vi "WPI_DashboardLog NetworkTables.vi"(8 "Occasional DB Data":T1, 9 "Frequent DB Data":T2, 11 "NT Data Values":T7(array[cluster])) -> ()   [LabVIEW 2017]
uses:
  <vilib>/Rock Robotics/Network Tables/Protocol Operations.ctl
  <vilib>/Rock Robotics/Network Tables/Field Data.ctl
  <vilib>/Rock Robotics/Network Tables/Field Type.ctl
  <vilib>/Rock Robotics/Network Tables/Sequence.ctl
  <vilib>/Rock Robotics/Network Tables/Make Table Operation.ctl
  <vilib>/Rock Robotics/WPI/Dashboard/WPI_DashboardLogging Global.vi
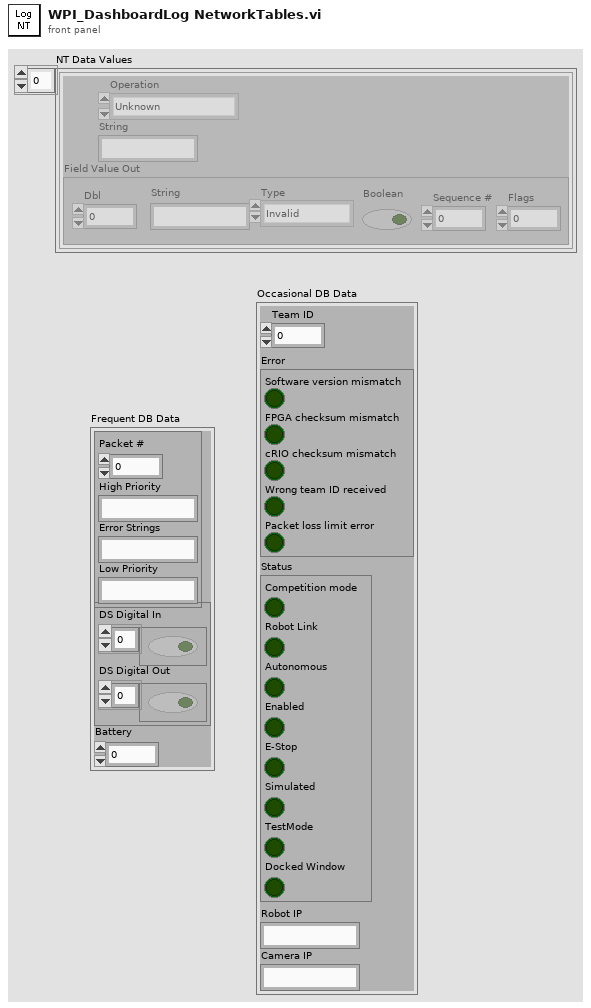
[diagram p1: front panel]
types:
  T1 = cluster{"Team ID":u16, "Error":cluster{"Software version mismatch":bool, "FPGA checksum mismatch":bool, "cRIO checksum mismatch":bool, "Wrong team ID received":bool, "Packet loss limit error":bool}, "Status":cluster{"Competition mode":bool, "Robot Link":bool, "Autonomous":bool, "Enabled":bool, "E-Stop":bool, "Simulated":bool, "TestMode":bool, "Docked Window":bool}, "Robot IP":string, "Camera IP":string}
  T2 = cluster{cluster{"Packet #":u8, "High Priority":string, "Error Strings":string, "Low Priority":string}, cluster{"DS Digital In":bool[], "DS Digital Out":bool[]}, "Battery":sgl}
  T3 = typedef "Protocol Operations.ctl" = enum16{"Unknown", "Keep Alive", "Client Hello", "Version not supported", "Server Hello Complete", "Assign", "Update", "No Op", "Server Hello", "Client Hello Complete", "Update Flags", "Delete Entry", "Delete All", "RPC Exec", "RPC Response"}
  T4 = typedef "Field Data.ctl" = cluster{"Dbl":dbl, "String":string, "Type":T5, "Boolean":bool, "Sequence #":T6, "Flags":u8}
  T5 = typedef "Field Type.ctl" = enum8{"Invalid", "Bool", "Numeric", "String", "Raw", "Boolean Array", "Numeric Array", "String Array", "RPC"}
  T6 = typedef "Sequence.ctl" = u16
  T7 = cluster{"Operation":T3, "String":string, "Field Value Out":T4}[]
  T8 = cluster{"size":u8, "tag":u8, "Version":cluster{"unsigned byte array[0]":u8, "unsigned byte array[1]":u8, "unsigned byte array[2]":u8, "unsigned byte array[3]":u8, "unsigned byte array[4]":u8, "unsigned byte array[5]":u8, "unsigned byte array[6]":u8, "unsigned byte array[7]":u8, "unsigned byte array[8]":u8, "unsigned byte array[9]":u8, "unsigned byte array[10]":u8}, "numPlayers":i8, "flags":u32, "floorClipPlane":cluster{"x":sgl, "y":sgl, "z":sgl, "w":sgl}, "Gravity Normal":cluster{"x":sgl, "y":sgl, "z":sgl}, "size":u8, "tag":u8, "Extra Data":cluster{"TrackingState":cluster{"TrackingState[0]":u8, "TrackingState[1]":u8, "TrackingState[2]":u8, "TrackingState[3]":u8, "TrackingState[4]":u8, "TrackingState[5]":u8, "TrackingState[6]":u8, "TrackingState[7]":u8, "TrackingState[8]":u8, "TrackingState[9]":u8, "TrackingState[10]":u8, "TrackingState[11]":u8, "TrackingState[12]":u8, "TrackingState[13]":u8, "TrackingState[14]":u8, "TrackingState[15]":u8, "TrackingState[16]":u8, "TrackingState[17]":u8, "TrackingState[18]":u8, "TrackingState[19]":u8}, "Position":cluster{"x":sgl, "y":sgl, "z":sgl}, "Quality":u32, "TrackState":enum32{"NotTracked", "PositionOnly", "Tracked"}}, "size":u8, "tag":u8, "Vertices":cluster{"Vertices[0]":cluster{"x":sgl, "y":sgl, "z":sgl}, "Vertices[1]":cluster{"x":sgl, "y":sgl, "z":sgl}, "Vertices[2]":cluster{"x":sgl, "y":sgl, "z":sgl}, "Vertices[3]":cluster{"x":sgl, "y":sgl, "z":sgl}, "Vertices[4]":cluster{"x":sgl, "y":sgl, "z":sgl}, "Vertices[5]":cluster{"x":sgl, "y":sgl, "z":sgl}, "Vertices[6]":cluster{"x":sgl, "y":sgl, "z":sgl}, "Vertices[7]":cluster{"x":sgl, "y":sgl, "z":sgl}, "Vertices[8]":cluster{"x":sgl, "y":sgl, "z":sgl}, "Vertices[9]":cluster{"x":sgl, "y":sgl, "z":sgl}, "Vertices[10]":cluster{"x":sgl, "y":sgl, "z":sgl}, "Vertices[11]":cluster{"x":sgl, "y":sgl, "z":sgl}, "Vertices[12]":cluster{"x":sgl, "y":sgl, "z":sgl}, "Vertices[13]":cluster{"x":sgl, "y":sgl, "z":sgl}, "Vertices[14]":cluster{"x":sgl, "y":sgl, "z":sgl}, "Vertices[15]":cluster{"x":sgl, "y":sgl, "z":sgl}, "Vertices[16]":cluster{"x":sgl, "y":sgl, "z":sgl}, "Vertices[17]":cluster{"x":sgl, "y":sgl, "z":sgl}, "Vertices[18]":cluster{"x":sgl, "y":sgl, "z":sgl}, "Vertices[19]":cluster{"x":sgl, "y":sgl, "z":sgl}}, "size":u8, "tag":u8, "Joystick":cluster{"axis 1":i8, "axis 2":i8, "axis 3":i8, "axis 4":i8, "axis 5":i8, "axis 6":i8, "Buttons":u16}, "Joystick 2":cluster{"axis 1":i8, "axis 2":i8, "axis 3":i8, "axis 4":i8, "axis 5":i8, "axis 6":i8, "Buttons":u16}, "size":u8, "tag":u8, "Custom Data":string}[]
  T9 = typedef "Make Table Operation.ctl" = enum16{"Get or Add Field", "Get Field or Add Temp", "Replace Temp ID", "Get Field ID - No Add", "Get Table Field IDs", "Get Field ID Info", "Move Field to Temp", "Validate", "Remove Field", "Remove All"}
  T10 = enum16{"open", "replace", "create", "open or create", "replace or create", "replace or create with confirmation"}
  T11 = cluster{"Operation":T3, "Name":string, "Field Value":T4}[]
  T12 = cluster{cluster{"High Priority":string, "Error Strings":string, "Low Priority":string}, cluster{u8, u8}, "Battery":sgl}
  T13 = cluster{"Team ID":u16, "Error":cluster{"Software version mismatch":bool, "FPGA checksum mismatch":bool, "cRIO checksum mismatch":bool, "Wrong team ID received":bool, "Packet loss limit error":bool}, "Status":cluster{"Competition mode":bool, "Robot Link":bool, "Autonomous":bool, "Enabled":bool, "E-Stop":bool, "Simulated":bool, "TestMode":bool, "Docked Window":bool}, "Robot IP":string, "Camera IP":string}[]
  T14 = cluster{"Video 1":i32, "Video 2":i32, "Video 3":i32, "Video 4":i32}
  T15 = cluster{i32, "Video Frame #":cluster{"Video 1":i32, "Video 2":i32, "Video 3":i32, "Video 4":i32}, "Logged Data":cluster{cluster{"High Priority":string, "Error Strings":string, "Low Priority":string}, cluster{u8, u8}, "Battery":sgl}, "Updates out":cluster{"Operation":T3, "Name":string, "Field Value":T4}[], cluster{"Team ID":u16, "Error":cluster{"Software version mismatch":bool, "FPGA checksum mismatch":bool, "cRIO checksum mismatch":bool, "Wrong team ID received":bool, "Packet loss limit error":bool}, "Status":cluster{"Competition mode":bool, "Robot Link":bool, "Autonomous":bool, "Enabled":bool, "E-Stop":bool, "Simulated":bool, "TestMode":bool, "Docked Window":bool}, "Robot IP":string, "Camera IP":string}[], "Kinect Data":cluster{"size":u8, "tag":u8, "Version":cluster{"unsigned byte array[0]":u8, "unsigned byte array[1]":u8, "unsigned byte array[2]":u8, "unsigned byte array[3]":u8, "unsigned byte array[4]":u8, "unsigned byte array[5]":u8, "unsigned byte array[6]":u8, "unsigned byte array[7]":u8, "unsigned byte array[8]":u8, "unsigned byte array[9]":u8, "unsigned byte array[10]":u8}, "numPlayers":i8, "flags":u32, "floorClipPlane":cluster{"x":sgl, "y":sgl, "z":sgl, "w":sgl}, "Gravity Normal":cluster{"x":sgl, "y":sgl, "z":sgl}, "size":u8, "tag":u8, "Extra Data":cluster{"TrackingState":cluster{"TrackingState[0]":u8, "TrackingState[1]":u8, "TrackingState[2]":u8, "TrackingState[3]":u8, "TrackingState[4]":u8, "TrackingState[5]":u8, "TrackingState[6]":u8, "TrackingState[7]":u8, "TrackingState[8]":u8, "TrackingState[9]":u8, "TrackingState[10]":u8, "TrackingState[11]":u8, "TrackingState[12]":u8, "TrackingState[13]":u8, "TrackingState[14]":u8, "TrackingState[15]":u8, "TrackingState[16]":u8, "TrackingState[17]":u8, "TrackingState[18]":u8, "TrackingState[19]":u8}, "Position":cluster{"x":sgl, "y":sgl, "z":sgl}, "Quality":u32, "TrackState":enum32{"NotTracked", "PositionOnly", "Tracked"}}, "size":u8, "tag":u8, "Vertices":cluster{"Vertices[0]":cluster{"x":sgl, "y":sgl, "z":sgl}, "Vertices[1]":cluster{"x":sgl, "y":sgl, "z":sgl}, "Vertices[2]":cluster{"x":sgl, "y":sgl, "z":sgl}, "Vertices[3]":cluster{"x":sgl, "y":sgl, "z":sgl}, "Vertices[4]":cluster{"x":sgl, "y":sgl, "z":sgl}, "Vertices[5]":cluster{"x":sgl, "y":sgl, "z":sgl}, "Vertices[6]":cluster{"x":sgl, "y":sgl, "z":sgl}, "Vertices[7]":cluster{"x":sgl, "y":sgl, "z":sgl}, "Vertices[8]":cluster{"x":sgl, "y":sgl, "z":sgl}, "Vertices[9]":cluster{"x":sgl, "y":sgl, "z":sgl}, "Vertices[10]":cluster{"x":sgl, "y":sgl, "z":sgl}, "Vertices[11]":cluster{"x":sgl, "y":sgl, "z":sgl}, "Vertices[12]":cluster{"x":sgl, "y":sgl, "z":sgl}, "Vertices[13]":cluster{"x":sgl, "y":sgl, "z":sgl}, "Vertices[14]":cluster{"x":sgl, "y":sgl, "z":sgl}, "Vertices[15]":cluster{"x":sgl, "y":sgl, "z":sgl}, "Vertices[16]":cluster{"x":sgl, "y":sgl, "z":sgl}, "Vertices[17]":cluster{"x":sgl, "y":sgl, "z":sgl}, "Vertices[18]":cluster{"x":sgl, "y":sgl, "z":sgl}, "Vertices[19]":cluster{"x":sgl, "y":sgl, "z":sgl}}, "size":u8, "tag":u8, "Joystick":cluster{"axis 1":i8, "axis 2":i8, "axis 3":i8, "axis 4":i8, "axis 5":i8, "axis 6":i8, "Buttons":u16}, "Joystick 2":cluster{"axis 1":i8, "axis 2":i8, "axis 3":i8, "axis 4":i8, "axis 5":i8, "axis 6":i8, "Buttons":u16}, "size":u8, "tag":u8, "Custom Data":string}[]}
  T16 = typedef "Field ID.ctl" = i32
  T17 = cluster{"Operation":T3, "String":string, "Field Value Out":T4}
  T18 = cluster{"Version":i32, "Duration":i32, "seconds since 1Jan1904":timestamp, "Robot IP":string}
  T19 = cluster{i32, i32, "Logged Data":cluster{cluster{"High Priority":string, "Error Strings":string, "Low Priority":string}, cluster{u8, u8}, "Battery":sgl}, "Updates out":cluster{"Operation":T3, "Name":string, "Field Value":T4}[], cluster{"Team ID":u16, "Error":cluster{"Software version mismatch":bool, "FPGA checksum mismatch":bool, "cRIO checksum mismatch":bool, "Wrong team ID received":bool, "Packet loss limit error":bool}, "Status":cluster{"Competition mode":bool, "Robot Link":bool, "Autonomous":bool, "Enabled":bool, "E-Stop":bool, "Simulated":bool, "TestMode":bool, "Docked Window":bool}, "Robot IP":string, "Camera IP":string}[], "Kinect Data":cluster{"size":u8, "tag":u8, "Version":cluster{"unsigned byte array[0]":u8, "unsigned byte array[1]":u8, "unsigned byte array[2]":u8, "unsigned byte array[3]":u8, "unsigned byte array[4]":u8, "unsigned byte array[5]":u8, "unsigned byte array[6]":u8, "unsigned byte array[7]":u8, "unsigned byte array[8]":u8, "unsigned byte array[9]":u8, "unsigned byte array[10]":u8}, "numPlayers":i8, "flags":u32, "floorClipPlane":cluster{"x":sgl, "y":sgl, "z":sgl, "w":sgl}, "Gravity Normal":cluster{"x":sgl, "y":sgl, "z":sgl}, "size":u8, "tag":u8, "Extra Data":cluster{"TrackingState":cluster{"TrackingState[0]":u8, "TrackingState[1]":u8, "TrackingState[2]":u8, "TrackingState[3]":u8, "TrackingState[4]":u8, "TrackingState[5]":u8, "TrackingState[6]":u8, "TrackingState[7]":u8, "TrackingState[8]":u8, "TrackingState[9]":u8, "TrackingState[10]":u8, "TrackingState[11]":u8, "TrackingState[12]":u8, "TrackingState[13]":u8, "TrackingState[14]":u8, "TrackingState[15]":u8, "TrackingState[16]":u8, "TrackingState[17]":u8, "TrackingState[18]":u8, "TrackingState[19]":u8}, "Position":cluster{"x":sgl, "y":sgl, "z":sgl}, "Quality":u32, "TrackState":enum32{"NotTracked", "PositionOnly", "Tracked"}}, "size":u8, "tag":u8, "Vertices":cluster{"Vertices[0]":cluster{"x":sgl, "y":sgl, "z":sgl}, "Vertices[1]":cluster{"x":sgl, "y":sgl, "z":sgl}, "Vertices[2]":cluster{"x":sgl, "y":sgl, "z":sgl}, "Vertices[3]":cluster{"x":sgl, "y":sgl, "z":sgl}, "Vertices[4]":cluster{"x":sgl, "y":sgl, "z":sgl}, "Vertices[5]":cluster{"x":sgl, "y":sgl, "z":sgl}, "Vertices[6]":cluster{"x":sgl, "y":sgl, "z":sgl}, "Vertices[7]":cluster{"x":sgl, "y":sgl, "z":sgl}, "Vertices[8]":cluster{"x":sgl, "y":sgl, "z":sgl}, "Vertices[9]":cluster{"x":sgl, "y":sgl, "z":sgl}, "Vertices[10]":cluster{"x":sgl, "y":sgl, "z":sgl}, "Vertices[11]":cluster{"x":sgl, "y":sgl, "z":sgl}, "Vertices[12]":cluster{"x":sgl, "y":sgl, "z":sgl}, "Vertices[13]":cluster{"x":sgl, "y":sgl, "z":sgl}, "Vertices[14]":cluster{"x":sgl, "y":sgl, "z":sgl}, "Vertices[15]":cluster{"x":sgl, "y":sgl, "z":sgl}, "Vertices[16]":cluster{"x":sgl, "y":sgl, "z":sgl}, "Vertices[17]":cluster{"x":sgl, "y":sgl, "z":sgl}, "Vertices[18]":cluster{"x":sgl, "y":sgl, "z":sgl}, "Vertices[19]":cluster{"x":sgl, "y":sgl, "z":sgl}}, "size":u8, "tag":u8, "Joystick":cluster{"axis 1":i8, "axis 2":i8, "axis 3":i8, "axis 4":i8, "axis 5":i8, "axis 6":i8, "Buttons":u16}, "Joystick 2":cluster{"axis 1":i8, "axis 2":i8, "axis 3":i8, "axis 4":i8, "axis 5":i8, "axis 6":i8, "Buttons":u16}, "size":u8, "tag":u8, "Custom Data":string}[]}
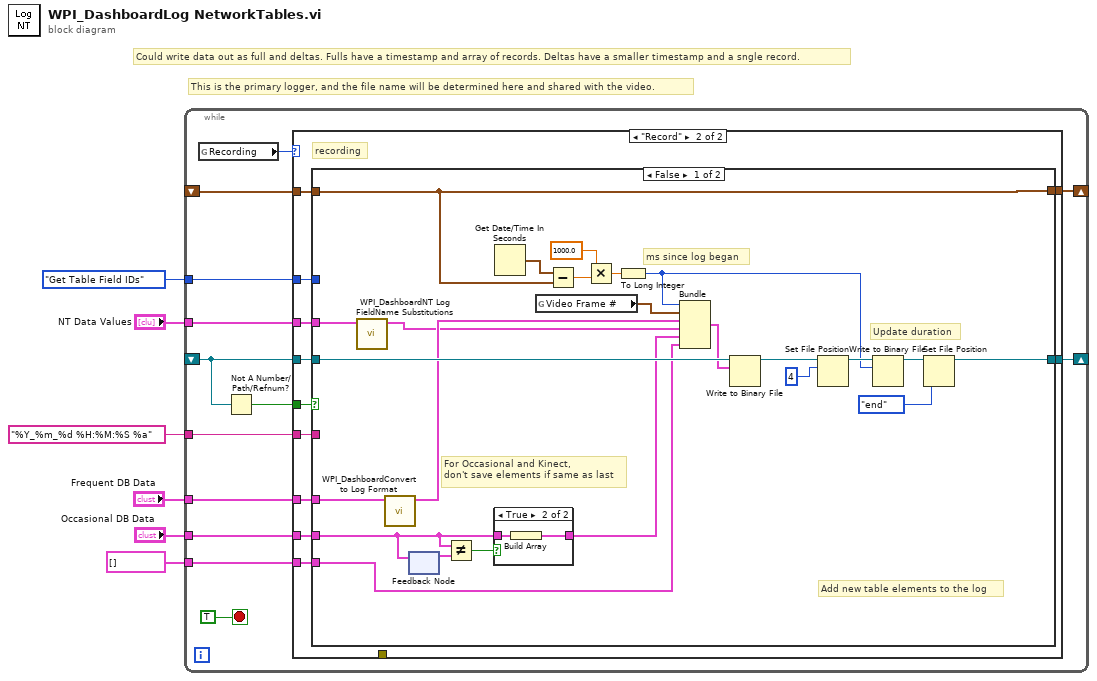
[diagram p0: block diagram]
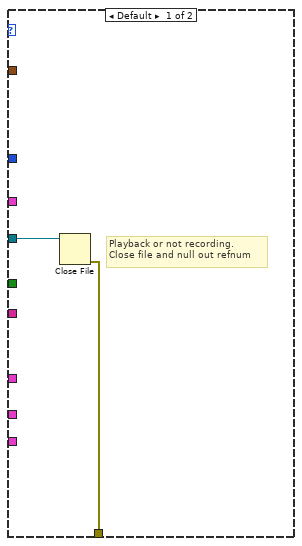
[diagram p2: hidden frame]
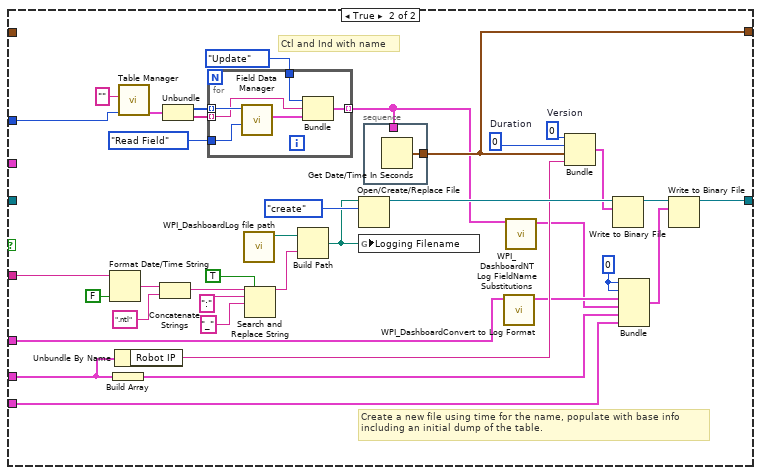
[diagram p4: hidden frame]
diagram:
  # "Could write data out as full and deltas. Fulls have a timestamp and array of records. Deltas have a smaller timestamp and a sngle record."
  # "This is the primary logger, and the file name will be determined here and shared with the video."
  n1 = while {
    shift-right: [w18] -> _
    shift-left: _ -> [w15]
    tunnel: Make_Table_Operation."Get Table Field IDs" ("Operation") -> [w17]
    tunnel: "NT Data Values" -> [w16]
    tunnel: "%Y_%m_%d %H:%M:%S %a" ("time format string (%c)") -> [w12]
    shift-right: [w11] -> _
    shift-left: _ -> [w10]
    tunnel: "Occasional DB Data" -> [w9]
    tunnel: "Frequent DB Data" -> [w8]
    tunnel: T8 [] ("Kinect Data") -> [w7]
    stop <- TRUE stop-if-true
    n2 = global read "WPI_DashboardLogging Global.vi" "Recording"() -> (w13:enum32{"Stop", "Record", "Playback"})
    n3 = Not A Number/Path/Refnum?(number/path/refnum=w15) -> (NaN/Path/Refnum?=w14:bool)
    n4 = case shown="\"Record\"" w13 {
      tunnel: [_ w32] -> w18
      tunnel: w17 -> [_ w31]
      tunnel: w16 -> [_ w30]
      tunnel: w15 -> [w21 w29]
      tunnel: w14 -> [_ w28]
      tunnel: w12 -> [_ w27]
      tunnel: [_ w26] -> w11
      tunnel: w10 -> [_ w25]
      tunnel: [w20 _] -> _
      tunnel: w9 -> [_ w24]
      tunnel: w8 -> [_ w23]
      tunnel: w7 -> [_ w22]
      frame Default {
        # "Playback or not recording.\nClose file and null out refnum"
        n5 = Close File(refnum=w21) -> (error out=w20:errorcluster)  [unwired: 1 in, 1 out]
      }
      frame "Record" {
        # "recording"
        n6 = case shown="False" w28 {
          tunnel: [w54 w72] -> w32
          tunnel: w31 -> [_ w84]
          tunnel: w29 -> [w56 _]
          tunnel: w30 -> [w35 _]
          tunnel: w27 -> [_ w81]
          tunnel: [w55 w69] -> w26
          tunnel: w25 -> [w55 _]
          tunnel: w24 -> [w39 w65]
          tunnel: w23 -> [w37 w63]
          tunnel: w22 -> [w33 w59]
          frame False {
            # "For Occasional and Kinect,\ndon't save elements if same as last"
            # "Update duration"
            # "ms since log began"
            # "Add new table elements to the log"
            n7 = call <vilib>:"WPI_DashboardNT Log FieldName Substitutions.vi"("Updates in"=w35) -> ("Updates out"=w34:T11)  [unwired: 10 in]
            n8 = call <vilib>:"WPI_DashboardConvert to Log Format.vi"("Frequent DB Data"=w37) -> ("Logged Data"=w36:T12)  [unwired: 10 in]
            n9 = feedback-in #1(w39) -> ()
            n10 = feedback #1() -> (w40:T1)  [unwired: 1 in]
            n11 = Not Equal?(x=w39, y=w40) -> (x != y?=w38:bool)
            n12 = case shown="True" w38 {
              tunnel: [_ w58] -> w41
              tunnel: w39 -> [_ w57]
              frame False {
              }
              frame True {
                n13 = Build Array(w57) -> (w58:T13)
              }
            }
            n14 = Get Date/Time In Seconds() -> (seconds since 1Jan1904=w51:timestamp)
            n15 = global read "WPI_DashboardLogging Global.vi" "Video Frame #"() -> (w52:T14)
            n16 = Subtract(x=w51, y=w55) -> (x-y=w50:dbl)
            n17 = Multiply(x=1000.0, y=w50) -> (x*y=w49:dbl)
            n18 = To Long Integer(number=w49) -> (32bit integer=w42:i32)
            n19 = Bundle(w42, "Video Frame #"=w52, "Logged Data"=w36, "Updates out"=w34, w41, "Kinect Data"=w33) -> (w53:T15)  [unwired: 1 in]
            n20 = Write to Binary File(file (use dialog)=w56, data=w53) -> (refnum out=w45:refnum<file>)  [unwired: 4 in, 2 out]
            n21 = Set File Position(offset (in bytes) (0)=i64 4, refnum=w45) -> (refnum out=w44:refnum<file>)  [unwired: 2 in, 1 out]
            n22 = Write to Binary File(file (use dialog)=w44, data=w42) -> (refnum out=w47:refnum<file>)  [unwired: 4 in, 2 out]
            n23 = Set File Position(refnum=w47, from (0:start)=enum16{"start", "end", "current"}."end") -> (refnum out=w54:refnum<file>)  [unwired: 2 in, 1 out]
          }
          frame True {
            w67 = 0  # Duration
            w70 = 0
            w68 = 0  # Version
            # "Create a new file using time for the name, populate with base info\nincluding an initial dump of the table."
            # "Ctl and Ind with name"
            n24 = Format Date/Time String(time format string (%c)=w81, UTC format=FALSE) -> (date/time string=w80:string)  [unwired: 1 in]
            n25 = Build Array(w65) -> (w64:T13)
            n26 = Unbundle By Name(w65) -> ("Robot IP"=w66:string)
            n27 = call <vilib>:"Table Manager.vi"("Operation"=w84, "Entry Name"="") -> ("Entries"=w92:cluster{"Entry IDs":T16[], "Names":string[]})  [unwired: 6 in, 3 out]
            n28 = Concatenate Strings(w80, ".ntl" ("time format string (%c)")) -> (w75:string)
            n29 = Unbundle(w92) -> ("Entry IDs"=w93:T16[], "Names"=w94:string[])
            n30 = for {
              tunnel: w93 -> [w100] mode=indexing
              tunnel: [w99] -> w60 mode=indexing
              tunnel: enum16{"Update Field", "Read Field"}."Read Field" ("Operation") -> [w101]
              tunnel: w94 -> [w98] mode=indexing
              tunnel: Protocol_Operations."Update" ("Operation") -> [w96]
              n31 = call <vilib>:"Field Data Manager.vi"("Operation"=w101, "Field ID"=w100) -> ("Field Value Out"=w97:T4)  [unwired: 8 in, 1 out]
              n32 = Bundle("Operation"=w96, "String"=w98, "Field Value Out"=w97) -> (w99:T17)  [unwired: 1 in]
            }
            n33 = call <vilib>:"WPI_DashboardLog file path.vi"() -> ("appended path"=w89:path)  [unwired: 11 in]
            n34 = Search and Replace String(replace all?=TRUE ("replace all? (F)"), input string=w75, search string=":", replace string="_") -> (result string=w74:string)  [unwired: 4 in, 3 out]
            n35 = Build Path(base path=w89, name or relative path=w74) -> (appended path=w83:path)
            n36 = Open/Create/Replace File(file path (use dialog)=w83, operation (0:open)=T10."create") -> (refnum out=w86:refnum<file>)  [unwired: 4 in, 2 out]
            n37 = global write "WPI_DashboardLogging Global.vi" "Logging Filename"(w83) -> ()
            n38 = stacked-sequence {
              tunnel: [w95] -> w69
              tunnel: w60 -> [_]
              frame #0 {
                n39 = Get Date/Time In Seconds() -> (seconds since 1Jan1904=w95:timestamp)
              }
            }
            n40 = call <vilib>:"WPI_DashboardConvert to Log Format.vi"("Frequent DB Data"=w63) -> ("Logged Data"=w62:T12)  [unwired: 10 in]
            n41 = call <vilib>:"WPI_DashboardNT Log FieldName Substitutions.vi"("Updates in"=w60) -> ("Updates out"=w61:T11)  [unwired: 10 in]
            n42 = Bundle("Version"=w68, "Duration"=w67, "seconds since 1Jan1904"=w69, "Robot IP"=w66) -> (w85:T18)  [unwired: 1 in]
            n43 = Write to Binary File(file (use dialog)=w86, data=w85) -> (refnum out=w73:refnum<file>)  [unwired: 4 in, 2 out]
            n44 = Bundle(w70, w70, "Logged Data"=w62, "Updates out"=w61, w64, "Kinect Data"=w59) -> (w71:T19)  [unwired: 1 in]
            n45 = Write to Binary File(file (use dialog)=w73, data=w71) -> (refnum out=w72:refnum<file>)  [unwired: 4 in, 2 out]
          }
        }
      }
    }
  }
